vi "NT Write String Array.vi"(4 "options":T1={"Send All"=FALSE, "Keep Duplicates"=FALSE, "rate (hz)"=10}, 6 "timestamp":u64, 8 "error in":errorcluster, 9 "value":string[](array[string]), 11 "name":string="String Array") -> (0 "error out":errorcluster)   [LabVIEW 2025]
doc: "Update the array of strings to the named topic."
uses:
  <vilib>/Rock Robotics/Network Tables/NT PublishOptions.ctl
  <vilib>/Rock Robotics/Network Tables/NT Datatype.ctl
panel:
  in  "description":string="string[]"
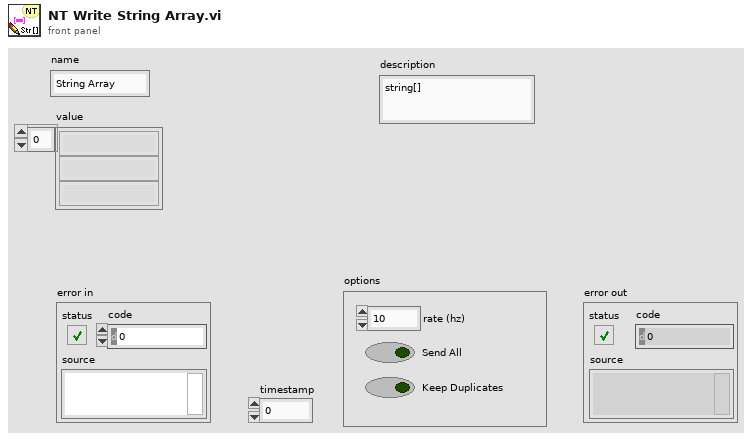
[diagram p1: front panel]
types:
  T1 = typedef "NT PublishOptions.ctl" = cluster{"Send All":bool, "Keep Duplicates":bool, "rate (hz)":u64}
  T2 = typedef "NT Datatype.ctl" = u32
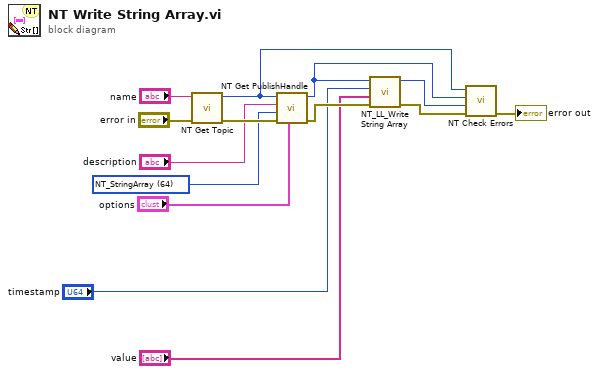
[diagram p0: block diagram]
diagram:
  w11 = T2 64 items=["NT_Unassigned"=0, "NT_Boolean"=1, "NT_Double"=2, "NT_String"=4, "NT_Raw"=8, "NT_BooleanArray"=16, "NT_DoubleArray"=32, "NT_StringArray"=64, "NT_RPC"=128, "NT_Integer"=256, "NT_Float"=512, "NT_IntegerArray"=1024, "NT_FloatArray"=2048] ("NT_Type")
  n1 = call <vilib>:"NT Get Topic.vi"("error in (no error)"="error in", "name"="name") -> ("error out"=w12:errorcluster, "topicHandle"=w4:u32)  [unwired: 8 in]
  n2 = call <vilib>:"NT Get PublishHandle.vi"("options"="options", "error in (no error)"=w12, "NT_Type"=w11, "description"="description", "topicHandle"=w4) -> ("error out"=w10:errorcluster, "publishHandle"=w3:u32)  [unwired: 5 in]
  n3 = call <vilib>:"NT_LL_Write String Array.vi"("error in (no error)"=w10, "value"="value", "timestamp"="timestamp", "publishHandle"=w3) -> ("error out"=w7:errorcluster, "success"=w2:u32)  [unwired: 6 in]
  n4 = call <vilib>:"NT Check Errors.vi"("error in (no error)"=w7, "success"=w2, "pubSubHandle"=w3, "topicHandle"=w4) -> ("error out"=→"error out":errorcluster)  [unwired: 7 in]
